vi "http write header to string.vi"(11 "application request":T1) -> (3 "header string":string)   [LabVIEW 2016, in "Basic HTTPS server.lvclass"]
uses:
  Basic HTTPS server.lvclass
  http response.ctl
  HTTP headers/http header data.ctl
  HTTP headers/http headers.lvlib
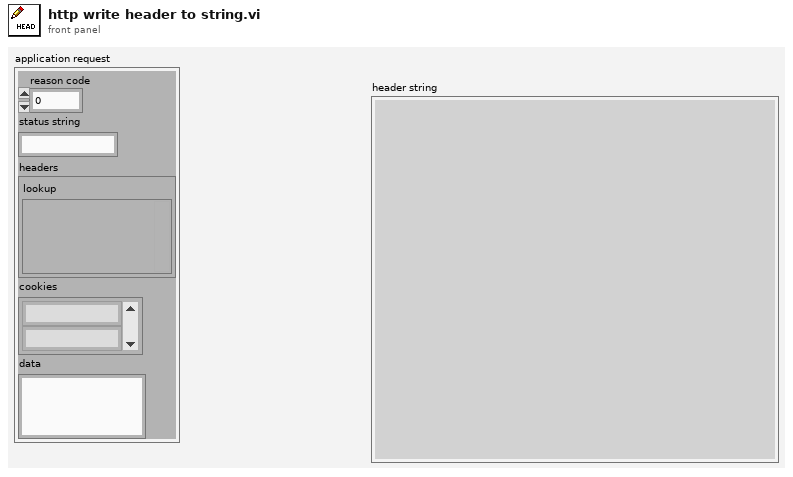
[diagram p1: front panel]
types:
  T1 = typedef "Basic HTTPS server.lvclass/http response.ctl" = cluster{"reason code":u16, "status string":string, "headers":T2, "cookies":string[], "data":string}
  T2 = typedef "http headers.lvlib/http header data.ctl" = cluster{"lookup":variant}
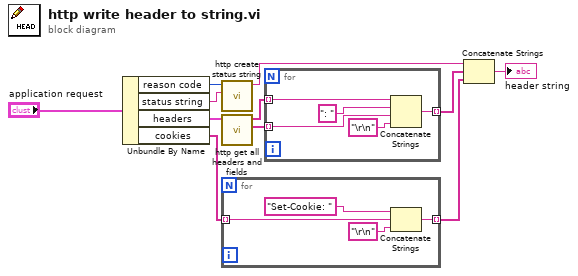
[diagram p0: block diagram]
diagram:
  n1 = Unbundle By Name("application request") -> ("reason code"=w8:u16, "status string"=w10:string, "headers"=w3:T2, "cookies"=w11:string[])
  n2 = call "http create status string.vi"("status string"=w10, "reason code"=w8) -> ("status line"=w7:string)  [unwired: 9 in]
  n3 = call "http get all headers and fields.vi"("headers"=w3) -> ("data"=w1:string[], "fields"=w2:string[])  [unwired: 9 in]
  n4 = for {
    tunnel: w11 -> [w13] mode=indexing
    tunnel: [w12] -> w5 mode=indexing
    n5 = Concatenate Strings("Set-Cookie: " ("string"), w13, "\r\n" ("format string")) -> (w12:string)
  }
  n6 = for {
    tunnel: w2 -> [w20] mode=indexing
    tunnel: w1 -> [w18] mode=indexing
    tunnel: [w16] -> w6 mode=indexing
    n7 = Concatenate Strings(w20, ": " ("string"), w18, "\r\n" ("format string")) -> (w16:string)
  }
  n8 = Concatenate Strings(w7, w6, w5) -> (→"header string":string)
